vi "set options.vi"(8 "error in":errorcluster, 10 "options":i32[](array[numeric]), 11 "connection creator in":refnum<class "connection creator.lvclass">) -> (0 "error out":errorcluster)   [LabVIEW 2016, in "connection creator.lvclass"]
uses:
  connection creator.lvclass
  connection creator.lvclass/connection creator.ctl
  dllwrapper/async tls dl.lvlib
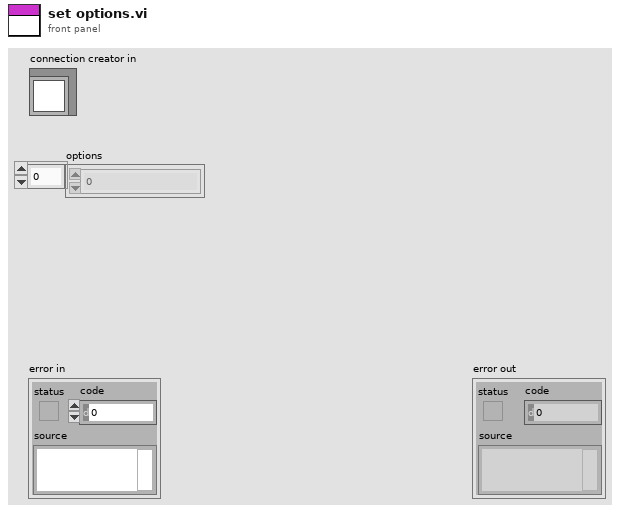
[diagram p1: front panel]
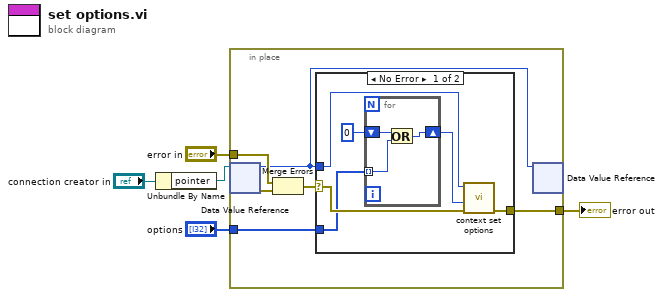
[diagram p0: block diagram]
diagram:
  n1 = Unbundle By Name("connection creator in") -> ("pointer"=w3:refnum<data-value>)
  n2 = in-place {
    in-place-border: "error in" -> [w10]
    in-place-border: [w8] -> w2
    in-place-border: "options" -> [w6]
    n3 = in-place-dvr #1(w3) -> (w7:u64, w11:errorcluster)
    n4 = Merge Errors(w10, w11) -> (w9:errorcluster)
    n5 = case shown="No Error" w9 {
      selector: w9 -> [w17 w21]
      tunnel: [w15 w21] -> w8
      tunnel: w7 -> [w16 _]
      tunnel: w6 -> [w12 _]
      frame No Error {
        n6 = for {
          shift-right: [w19] -> w13
          shift-left: 0 -> [w20]
          tunnel: w12 -> [w18] mode=indexing
          n7 = Or(x=w20, y=w18) -> (x .or. y?=w19:i32)
        }
        n8 = call "context set options.vi"("error in"=w17, "options"=w13, "connector"=w16) -> ("error out"=w15:errorcluster)  [unwired: 8 in]
      }
      frame Error {
      }
    }
    n9 = in-place-dvr #1(w7) -> ()  [unwired: 2 out]
  }
  "error out" <- w2
